vi "Lex Text-Comment.vi"(8 "Error In":errorcluster) -> (0 "Error Out":errorcluster)   [LabVIEW 2018, in "Tests.lvlib" / "Lexer.lvlib"]
uses:
  Lexer.lvlib
  src/Toolkit/Low-Level/Tokens/Text/Text.lvclass
  src/Toolkit/Low-Level/Tokens/Comment/Comment.lvclass
  <vilib>/addons/_JKI Toolkits/Caraya/classes/Assert/Assert Equal Type_Variant.vi
  src/Toolkit/Low-Level/Tokens/Contentable/Contentable.lvclass
  src/Toolkit/Low-Level/Lexer/Lexer.lvclass
  <vilib>/addons/_JKI Toolkits/Caraya/classes/Test/Test.lvclass
  <vilib>/addons/_JKI Toolkits/Caraya/classes/Assert/Assert.lvclass
  Tests.lvlib
  src/Toolkit/Low-Level/Tokens/Token/Token.lvclass
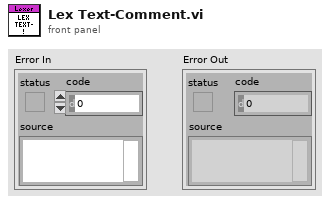
[diagram p1: front panel]
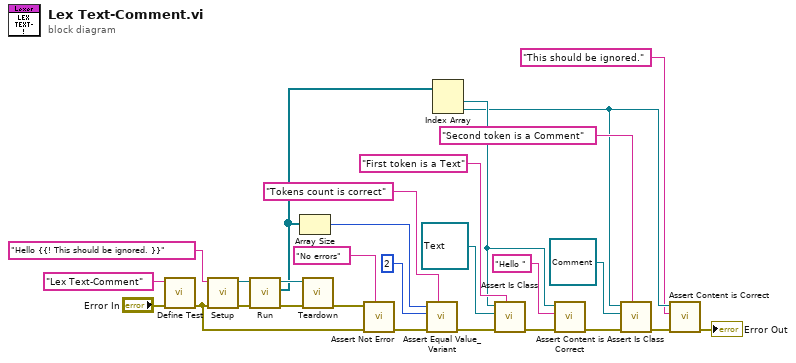
[diagram p0: block diagram]
diagram:
  n1 = call <vilib>:"Define Test.vi"("error in (no error)"="Error In", "Label (VI Title)"="Lex Text-Comment") -> ("error out"=w3:errorcluster)  [unwired: 9 in]
  n2 = call "Setup.vi"("Error In"=w3, "String"="Hello {{! This should be ignored. }}" ("format string")) -> ("Error Out"=w7:errorcluster, "Lexer"=w8:refnum<class "Lexer.lvclass">)  [unwired: 8 in]
  n3 = call-dynamic "Run.vi"("Error In"=w7, "Lexer In"=w8) -> ("Error Out"=w5:errorcluster, "Tokens"=w1:refnum<class "Token.lvclass">[], "Lexer Out"=w6:refnum<class "Lexer.lvclass">)  [unwired: 7 in]
  n4 = Array Size(array=w1) -> (size(s)=w23:i32)
  n5 = call "Teardown.vi"("Error In"=w5, "Lexer"=w6) -> ("Error Out"=w2:errorcluster)  [unwired: 9 in]
  n6 = call <vilib>:"Assert Not Error.vi"("Label"="No errors", "error in (no error)"=w3, "Not Error?"=w2) -> ("error out"=w25:errorcluster)  [unwired: 8 in]
  n7 = call <vilib>:"Assert Equal Value_Variant.vi"("Label"="Tokens count is correct", "error in (no error)"=w25, "Y"=2 ("size(s)"), "X"=w23) -> ("error out"=w21:errorcluster)  [unwired: 7 in]
  n8 = Index Array(array=w1) -> (element #1=w16:refnum<class "Token.lvclass">, element #2=w10:refnum<class "Token.lvclass">)  [unwired: 2 in]
  n9 = call "Assert Is Class.vi"("Label"="First token is a Text", "Error In"=w21, "Expected"=refnum<class "Text.lvclass"> refnum ("Mustache.lvlib:Tokens.lvlib:Text.lvclass"), "Actual"=w16) -> ("Error Out"=w20:errorcluster)  [unwired: 7 in]
  n10 = call "Assert Content is Correct.vi"("Error In"=w20, "Expected"="Hello ", "Token"=w16) -> ("Error Out"=w15:errorcluster)  [unwired: 8 in]
  n11 = call "Assert Is Class.vi"("Label"="Second token is a Comment", "Error In"=w15, "Expected"=refnum<class "Comment.lvclass"> refnum ("Toolkit.lvlib:Tokens.lvlib:Comment.lvclass"), "Actual"=w10) -> ("Error Out"=w14:errorcluster)  [unwired: 7 in]
  n12 = call "Assert Content is Correct.vi"("Error In"=w14, "Expected"="This should be ignored.", "Token"=w10) -> ("Error Out"=→"Error Out":errorcluster)  [unwired: 8 in]
